vi "TeirToSensor.vi"(5 "Teir":T1) -> (0 "CL":dbl=3.0, 1 "CR":dbl=12.0, 2 "Teir Height":dbl=25.0)   [LabVIEW 2014, in "Elevator System.lvlib"]
uses:
  Elevator System.lvlib
  Typedef/TeirNumber.ctl
panel:
  in  "Tab Control":enum32{"Competition", "Simulation"}(tab)
  in  "Competition Settings":T2={"T1 Point"=6.0, "Delta"=17.0, "CR"=12.0, "CL"=3.0} {"CL" format="%#_13g"; "CR" format="%#_13g"; "Delta" format="%#_13g"; "T1 Point" format="%#_13g"}
  in  "Simulation Settings":T2={"T1 Point"=6.0, "Delta"=17.0, "CR"=12.0, "CL"=3.0} {"CL" format="%#_13g"; "CR" format="%#_13g"; "Delta" format="%#_13g"; "T1 Point" format="%#_13g"}
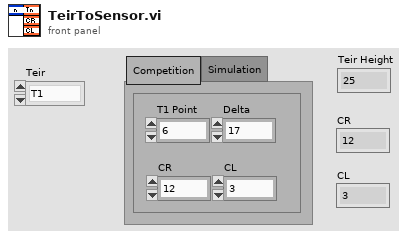
[diagram p1: front panel]
types:
  T1 = typedef "Elevator System.lvlib/TeirNumber.ctl" = enum16{"T1", "T2", "T3", "T4", "T5", "T6"}
  T2 = cluster{"T1 Point":dbl, "Delta":dbl, "CR":dbl, "CL":dbl}
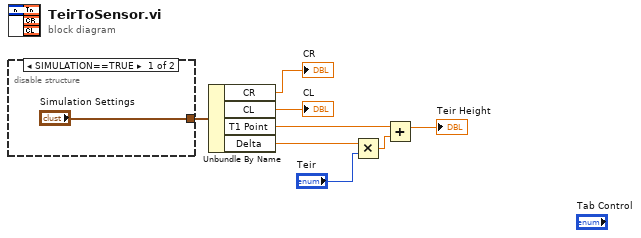
[diagram p0: block diagram]
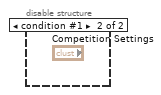
[diagram p2: hidden frame]
diagram:
  n1 = disable-structure shown="SIMULATION==TRUE" {
    disable-tunnel: ["Simulation Settings" _] -> w6
    frame condition #0 (active) {
    }
    frame condition #1 {
    }
  }
  n2 = Unbundle By Name(w6) -> ("CR"=→"CR":dbl, "CL"=→"CL":dbl, "T1 Point"=w3:dbl, "Delta"=w4:dbl)
  n3 = Multiply(x=w4, y="Teir") -> (x*y=w8:dbl)
  n4 = Add(x=w3, y=w8) -> (x+y=→"Teir Height":dbl)
